vi "Choose_tags.vi"(0 "Number of tags to read from":i32, 1 "mode":T1(ring)) -> (2 "Tags opened":string[](array[string]), 3 "Opened tags refnumbers":refnum<k13>[](array[refnum]), 4 "error out":errorcluster)   [LabVIEW 2023]
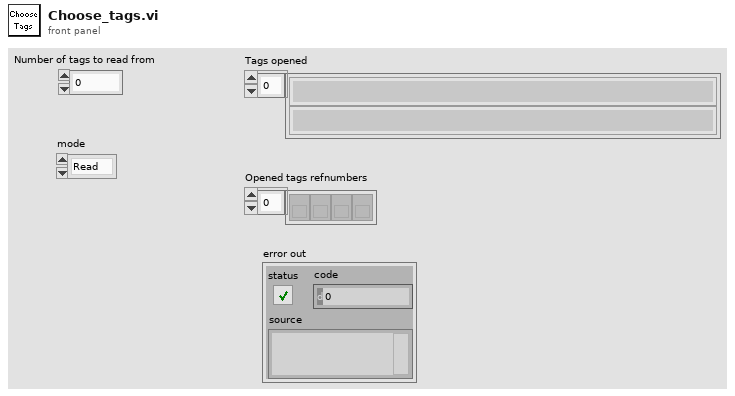
[diagram p1: front panel]
types:
  T1 = enum16{"Read", "Write", "ReadWrite", "BufferedRead", "BufferedReadWrite"}
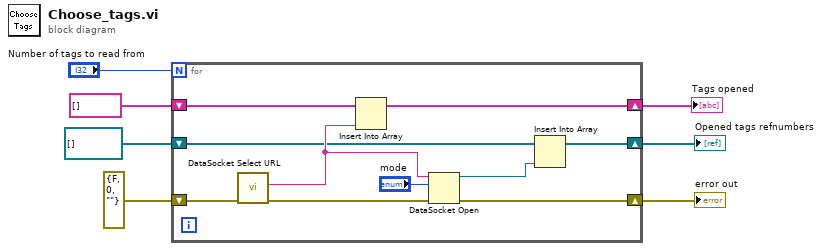
[diagram p0: block diagram]
diagram:
  n1 = for {
    N: "Number of tags to read from" -> [_]
    shift-right: [w16] -> w7
    shift-left: string[] [] -> [w17]
    shift-right: [w12] -> w5
    shift-left: errorcluster {"status"=FALSE, "code"=0, "source"=""} ("error out") -> [w15]
    shift-right: [w9] -> w4
    shift-left: refnum<k13>[] [] -> [w10]
    n2 = call <vilib>:"DataSocket Select URL.vi"("error in (no error)"=w15) -> ("error out"=w13:errorcluster, "URL"=w11:string)  [unwired: 8 in, 1 out]
    n3 = Insert Into Array "Insert Into Array"(array=w17, new element=w11) -> (w16:string[])  [unwired: 1 in]
    n4 = DataSocket Open(8:w13, 10:"mode", 11:w11) -> (0:w12:errorcluster, 3:w8:refnum<k13>)  [unwired: 1 in]
    n5 = Insert Into Array "Insert Into Array"(array=w10, new element=w8) -> (w9:refnum<k13>[])  [unwired: 1 in]
  }
  "Tags opened" <- w7
  "error out" <- w5
  "Opened tags refnumbers" <- w4
